vi "DriveForTime.vi"(10 "speed":dbl) -> ()   [LabVIEW 2020]
uses:
  <vilib>/Rock Robotics/WPI/ThirdParty/REV Robotics/REVLib/Typedef/Spark MAX Control Type.ctl
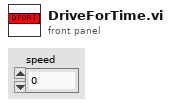
[diagram p1: front panel]
types:
  T1 = typedef "Spark MAX Control Type.ctl" = enum16{"Percent VBus", "Voltage", "Velocity", "Position", "Smart Motion", "Current", "Smart Velocity"}
  T2 = typedef "WPI_MotorControlDeviceRef.ctl" = cluster{"DeviceStatus":errorcluster, "Type":T3, "PWM":cluster{"PWM Channel":T4, "DeadBand":T5}, "CAN":cluster{"Device Number":u8, "SetOutput VI Ref":variant, "GetOutput VI Ref":variant, "Enable VI Ref":variant, "Disable VI Ref":variant, "Data":variant}, "Invert":bool, "DIO PWM":cluster{"PWM \"Enable\" Channel":T4, "DIOChannel":T6, "PWM Rate":dbl}}
  T3 = typedef "WPI_MotorControlType.ctl" = enum16{"PWM", "CAN", "DIO PWM"}
  T4 = typedef "FPGA_DIOPWMChannel.ctl" = enum8{"PWM 0", "PWM 1", "PWM 2", "PWM 3", "PWM 4", "PWM 5", "PWM 6", "PWM 7", "PWM 8", "PWM 9", "PWM MXP 0", "PWM MXP 1", "PWM MXP 2", "PWM MXP 3", "PWM MXP 4", "PWM MXP 5", "PWM MXP 6", "PWM MXP 7", "PWM MXP 8", "PWM MXP 9", "Invalid"}
  T5 = typedef "WPI_PWMDeadband.ctl" = cluster{"Name":string, "maxPositivePwm":i32, "minPositivePwm":i32, "centerPwm":i32, "maxNegativePwm":i32, "minNegativePwm":i32, "angularRange":u16}
  T6 = typedef "FPGA_DIOChannel.ctl" = enum8{"DIO 0", "DIO 1", "DIO 2", "DIO 3", "DIO 4", "DIO 5", "DIO 6", "DIO 7", "DIO 8", "DIO 9", "DIO MXP 0", "DIO MXP 1", "DIO MXP 2", "DIO MXP 3", "DIO MXP 4", "DIO MXP 5", "DIO MXP 6", "DIO MXP 7", "DIO MXP 8", "DIO MXP 9", "DIO MXP 10", "DIO MXP 11", "DIO MXP 12", "DIO MXP 13", "DIO MXP 14", "DIO MXP 15", "SPI Port CS1", "SPI Port CS2", "SPI Port CS3", "SPI Port MISO", "SPI Port MOSI", "Invalid"}
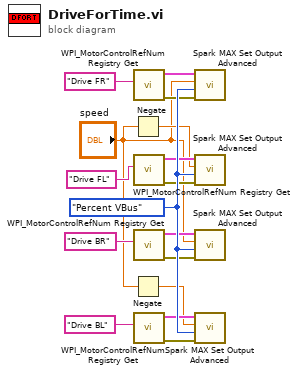
[diagram p0: block diagram]
diagram:
  w16 = Spark_MAX_Control_Type."Percent VBus" ("Control Mode")
  n1 = Negate(x="speed") -> (-x=w3:dbl)
  n2 = Negate(x="speed") -> (-x=w2:dbl)
  n3 = call <vilib>:"WPI_MotorControlRefNum Registry Get.vi"("refnum name"="Drive FR") -> ("error out"=w14:errorcluster, "MotorControlDevRef"=w15:T2)  [unwired: 9 in]
  n4 = call <vilib>:"WPI_MotorControlRefNum Registry Get.vi"("refnum name"="Drive FL") -> ("error out"=w12:errorcluster, "MotorControlDevRef"=w13:T2)  [unwired: 9 in]
  n5 = call <vilib>:"WPI_MotorControlRefNum Registry Get.vi"("refnum name"="Drive BR") -> ("error out"=w10:errorcluster, "MotorControlDevRef"=w11:T2)  [unwired: 9 in]
  n6 = call <vilib>:"WPI_MotorControlRefNum Registry Get.vi"("refnum name"="Drive BL") -> ("error out"=w8:errorcluster, "MotorControlDevRef"=w9:T2)  [unwired: 9 in]
  n7 = call <vilib>:"Spark MAX Set Output Advanced.vi"("error in (no error)"=w14, "Control Mode"=w16, "Setpoint"="speed", "MotorControlDevRef"=w15) -> ()  [unwired: 6 in, 2 out]
  n8 = call <vilib>:"Spark MAX Set Output Advanced.vi"("error in (no error)"=w12, "Control Mode"=w16, "Setpoint"=w3, "MotorControlDevRef"=w13) -> ()  [unwired: 6 in, 2 out]
  n9 = call <vilib>:"Spark MAX Set Output Advanced.vi"("error in (no error)"=w10, "Control Mode"=w16, "Setpoint"="speed", "MotorControlDevRef"=w11) -> ()  [unwired: 6 in, 2 out]
  n10 = call <vilib>:"Spark MAX Set Output Advanced.vi"("error in (no error)"=w8, "Control Mode"=w16, "Setpoint"=w2, "MotorControlDevRef"=w9) -> ()  [unwired: 6 in, 2 out]
